vi "ukol2.vi"() -> ()   [LabVIEW 2022 SP3]
panel:
  out "Numeric":i32
  out "Array 2":i32[](array[numeric])
  out "Array":u8[](array[numeric])
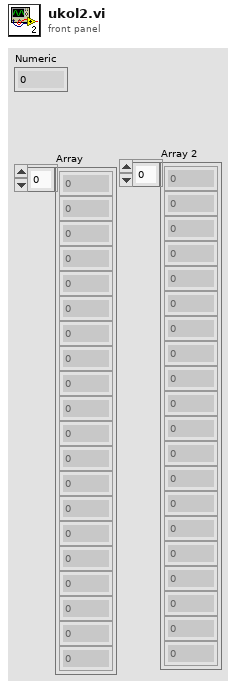
[diagram p1: front panel]
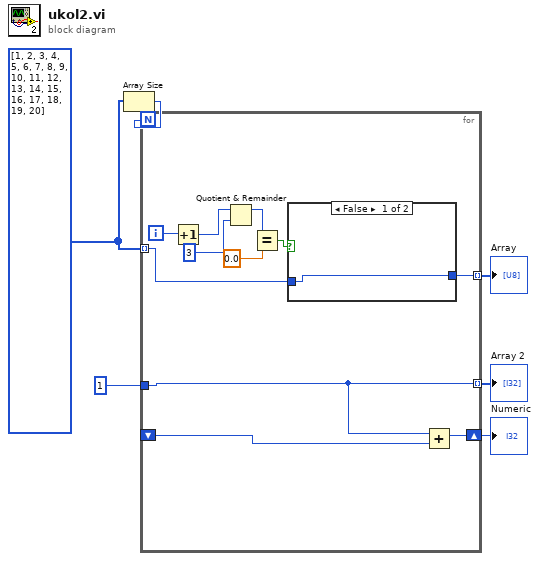
[diagram p0: block diagram]
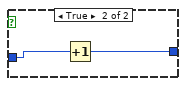
[diagram p2: hidden frame]
diagram:
  w4 = u8[] [1, 2, 3, 4, 5, 6, 7, 8, 9, 10, 11, 12, 13, 14, 15, 16, 17, 18, 19, 20]
  n1 = Array Size(array=w4) -> (size(s)=w6:i32)
  n2 = for {
    N: w6 -> [_]
    tunnel: w4 -> [w11] mode=indexing
    tunnel: [w10] -> w5 mode=indexing
    tunnel: 1 -> [w8]
    tunnel: [w8] -> w2 mode=indexing
    shift-right: [w9] -> w1
    shift-left: _ -> [w7]
    i -> [w17]
    n3 = Increment(x=w17) -> (x+1=w14:i32)
    n4 = Quotient & Remainder(x=w14, y=3) -> (x-y*floor(x/y)=w12:i32)  [unwired: 1 out]
    n5 = Equal?(x=w12, y=0.0) -> (x = y?=w15:bool)
    n6 = case shown="False" w15 {
      tunnel: w11 -> [w18 w20]
      tunnel: [w18 w19] -> w10
      frame False {
      }
      frame True {
        n7 = Increment(x=w20) -> (x+1=w19:u8)
      }
    }
    n8 = Add(x=w8, y=w7) -> (x+y=w9:i32)
  }
  "Array" <- w5
  "Array 2" <- w2
  "Numeric" <- w1
